vi "Create Timing (cluster).vi"(8 "error in (no error)":errorcluster, 11 "cycle timing":T1) -> (0 "error out":errorcluster, 3 "Timing":refnum<class "Timing.lvclass">)   [LabVIEW 2017, in "DSF Core.lvlib" / "Timing.lvclass"]
uses:
  Timing.lvclass
  DSF Configuration API/Public/Controls/DSF Timing Info.ctl
  Timing.lvclass/Timing.ctl
  Invalid Offset.vi
  Invalid Priority.vi
  DSF Core.lvlib
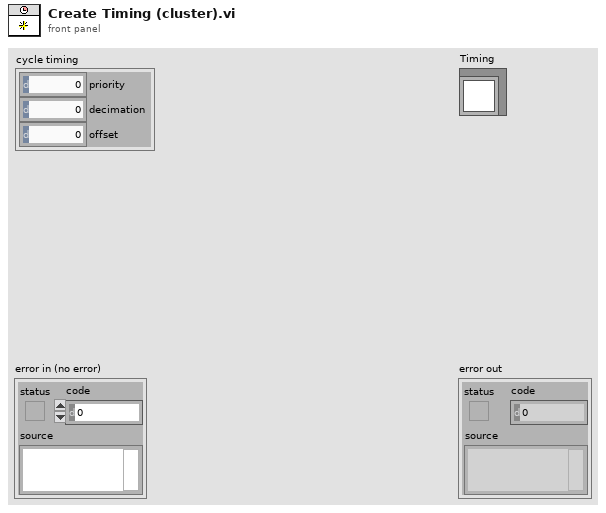
[diagram p1: front panel]
types:
  T1 = typedef "DSF Core.lvlib/DSF Timing Info.ctl" = cluster{"priority":u64, "decimation":u64, "offset":u64}
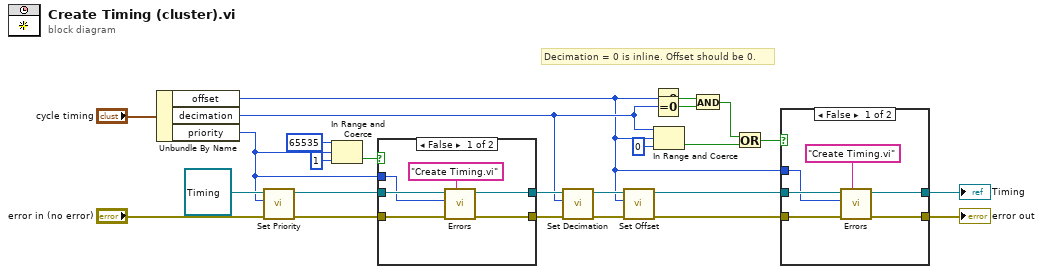
[diagram p0: block diagram]
diagram:
  # "Decimation = 0 is inline. Offset should be 0."
  n1 = Unbundle By Name("cycle timing") -> ("offset"=w2:u64, "decimation"=w3:u64, "priority"=w4:u64)
  n2 = call "Set Priority.vi"("Priority"=w4, "Timing in"=refnum<class "Timing.lvclass"> refnum ("Timing")) -> ("Timing out"=w11:refnum<class "Timing.lvclass">)  [unwired: 9 in]
  n3 = In Range and Coerce(upper limit=u64 65535, x=w4, lower limit=u64 1) -> (In Range?=w5:bool)  [unwired: 1 out]
  n4 = case shown="False" w5 {
    tunnel: w11 -> [w28 w30]
    tunnel: [w27 w30] -> w10
    tunnel: "error in (no error)" -> [w26 w29]
    tunnel: [w25 w29] -> w8
    tunnel: w4 -> [w23 _]
    frame False {
      n5 = call-poly "Errors.vi"("error source vi name"="Create Timing.vi", "error in (no error)"=w26, "priority"=w23, "Timing in"=w28) -> ("error out"=w25:errorcluster, "Timing out"=w27:refnum<class "Timing.lvclass">)  [unwired: 6 in]
    }
    frame True {
    }
  }
  n6 = call "Set Decimation.vi"("Decimation"=w3, "Timing in"=w10) -> ("Timing out"=w21:refnum<class "Timing.lvclass">)  [unwired: 9 in]
  n7 = call "Set Offset.vi"("Offset"=w2, "Timing in"=w21) -> ("Timing out"=w19:refnum<class "Timing.lvclass">)  [unwired: 9 in]
  n8 = Equal To 0?(x=w2) -> (x = 0?=w15:bool)
  n9 = Equal To 0?(x=w3) -> (x = 0?=w16:bool)
  n10 = In Range and Coerce(upper limit=w3, x=w2, lower limit=u64 0) -> (In Range?=w14:bool)  [unwired: 1 out]
  n11 = And(x=w15, y=w16) -> (x .and. y?=w12:bool)
  n12 = Or(x=w12, y=w14) -> (x .or. y?=w13:bool)
  n13 = case shown="False" w13 {
    tunnel: w19 -> [w36 w38]
    tunnel: [w35 w38] -> w18
    tunnel: [w34 w37] -> w17
    tunnel: w8 -> [w33 w37]
    tunnel: w2 -> [w32 _]
    frame False {
      n14 = call-poly "Errors.vi"("error source vi name"="Create Timing.vi", "error in (no error)"=w33, "offset"=w32, "Timing in"=w36) -> ("error out"=w34:errorcluster, "Timing out"=w35:refnum<class "Timing.lvclass">)  [unwired: 6 in]
    }
    frame True {
    }
  }
  "error out" <- w17
  "Timing" <- w18
